vi "Execute Message.vi"(8 "error in (no error)":errorcluster, 9 "timeout in ms (-1)":i32=-1, 11 "Abstract Consumer in":refnum<class "Abstract Consumer.lvclass">) -> (0 "error out":errorcluster, 1 "timed out?":bool, 2 "Stop?":bool, 3 "Abstract Consumer out":refnum<class "Abstract Consumer.lvclass">)   [LabVIEW 2027, in "Messaging.lvlib" / "Abstract Consumer.lvclass"]
uses:
  Abstract Consumer.lvclass
  Abstract Consumer.lvclass/Abstract Consumer.ctl
  Message/Abstract Request Message/Abstract Request Message.lvclass
  Message/Abstract Response Message/Abstract Response Message.lvclass
  Message Queue/Abstract Message Queue/Abstract Message Queue.lvclass
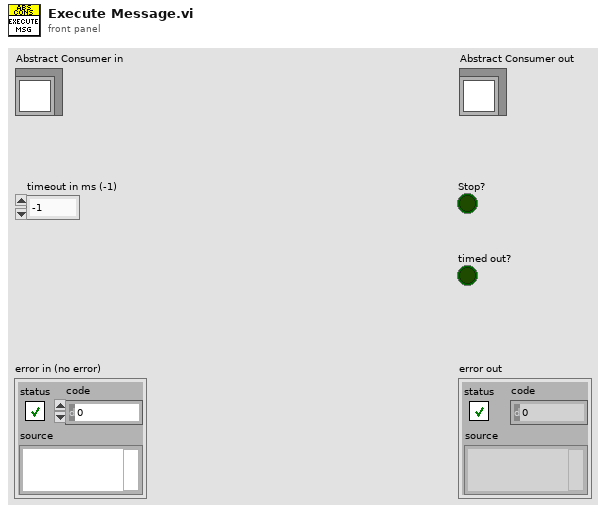
[diagram p1: front panel]
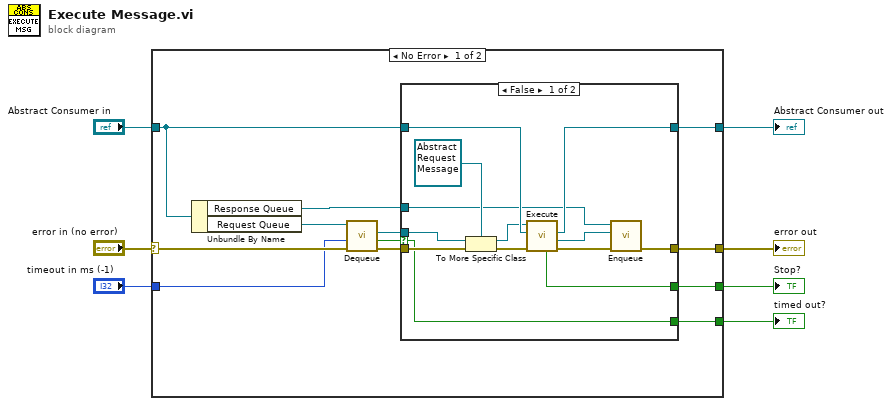
[diagram p0: block diagram]
diagram:
  n1 = case shown="No Error" "error in (no error)" {
    selector: "error in (no error)" -> [w18 w37]
    tunnel: [w17 w37] -> w6
    tunnel: [w15 w36] -> w4
    tunnel: "Abstract Consumer in" -> [w16 w36]
    tunnel: [w12 _] -> w3
    tunnel: "timeout in ms (-1)" -> [w11 _]
    tunnel: [w8 _] -> w1
    frame No Error {
      n2 = Unbundle By Name(w16) -> ("Response Queue"=w9:refnum<class "Abstract Message Queue.lvclass">, "Request Queue"=w19:refnum<class "Abstract Message Queue.lvclass">)
      n3 = call-dynamic "Dequeue.vi"("error in (no error)"=w18, "timeout in ms (-1)"=w11, "Abstract Message Queue in"=w19) -> ("error out"=w13:errorcluster, "timed out?"=w10:bool, "Message out"=w14:refnum<class "Abstract Message.lvclass">)  [unwired: 5 in, 1 out]
      n4 = case shown="False" w10 {
        selector: w10 -> [w20 w33]
        tunnel: [w23 w35] -> w17
        tunnel: w16 -> [w32 w34]
        tunnel: [w31 w34] -> w15
        tunnel: w14 -> [w29 _]
        tunnel: w13 -> [w27 w35]
        tunnel: [w25 _] -> w12
        tunnel: w9 -> [w22 _]
        tunnel: [w20 w33] -> w8
        frame False {
          n5 = To More Specific Class(target class=refnum<class "Abstract Request Message.lvclass"> refnum ("Message Queue Library.lvlib:Abstract Request Message.lvclass"), reference=w29, error in=w27) -> (specific class reference=w30:refnum<class "Abstract Request Message.lvclass">, error out=w26:errorcluster)
          n6 = call-dynamic "Execute.vi"("error in (no error)"=w26, "Abstract Consumer in"=w32, "Abstract Request Message in"=w30) -> ("error out"=w24:errorcluster, "Abstract Response out"=w21:refnum<class "Abstract Response Message.lvclass">, "Abstract Consumer out"=w31:refnum<class "Abstract Consumer.lvclass">, "Stop?"=w25:bool)  [unwired: 4 in, 1 out]
          n7 = call-dynamic "Enqueue.vi"("error in (no error)"=w24, "Message in"=w21, "Abstract Message Queue in"=w22) -> ("error out"=w23:errorcluster)  [unwired: 7 in, 1 out]
        }
        frame True {
        }
      }
    }
    frame Error {
    }
  }
  "error out" <- w6
  "Abstract Consumer out" <- w4
  "Stop?" <- w3
  "timed out?" <- w1
